vi "Pump_statusrequest.vi"(8 "error in (no error)":errorcluster, 10 "Command":string, 11 "VISA resource name":refnum<visa-resource-name>) -> (0 "error out":errorcluster, 1 "Message":string, 2 "Ready":bool, 3 "VISA resource name Out":refnum<visa-resource-name>, 4 "unsigned byte array":u8[](array[numeric]), 6 "Boolean array":bool[](array[boolean]))   [LabVIEW 2024]
uses:
  ab3bbe5a-7c2c-441d-9bf7-38fddc6173b4.vi
panel:
  out "Error present":bool
  out "read buffer":string
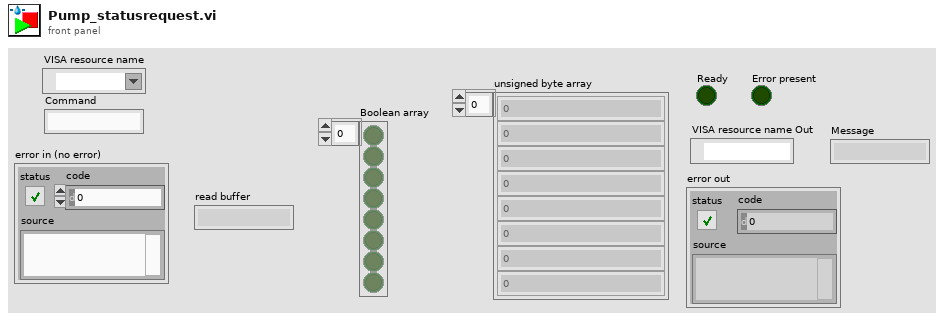
[diagram p1: front panel]
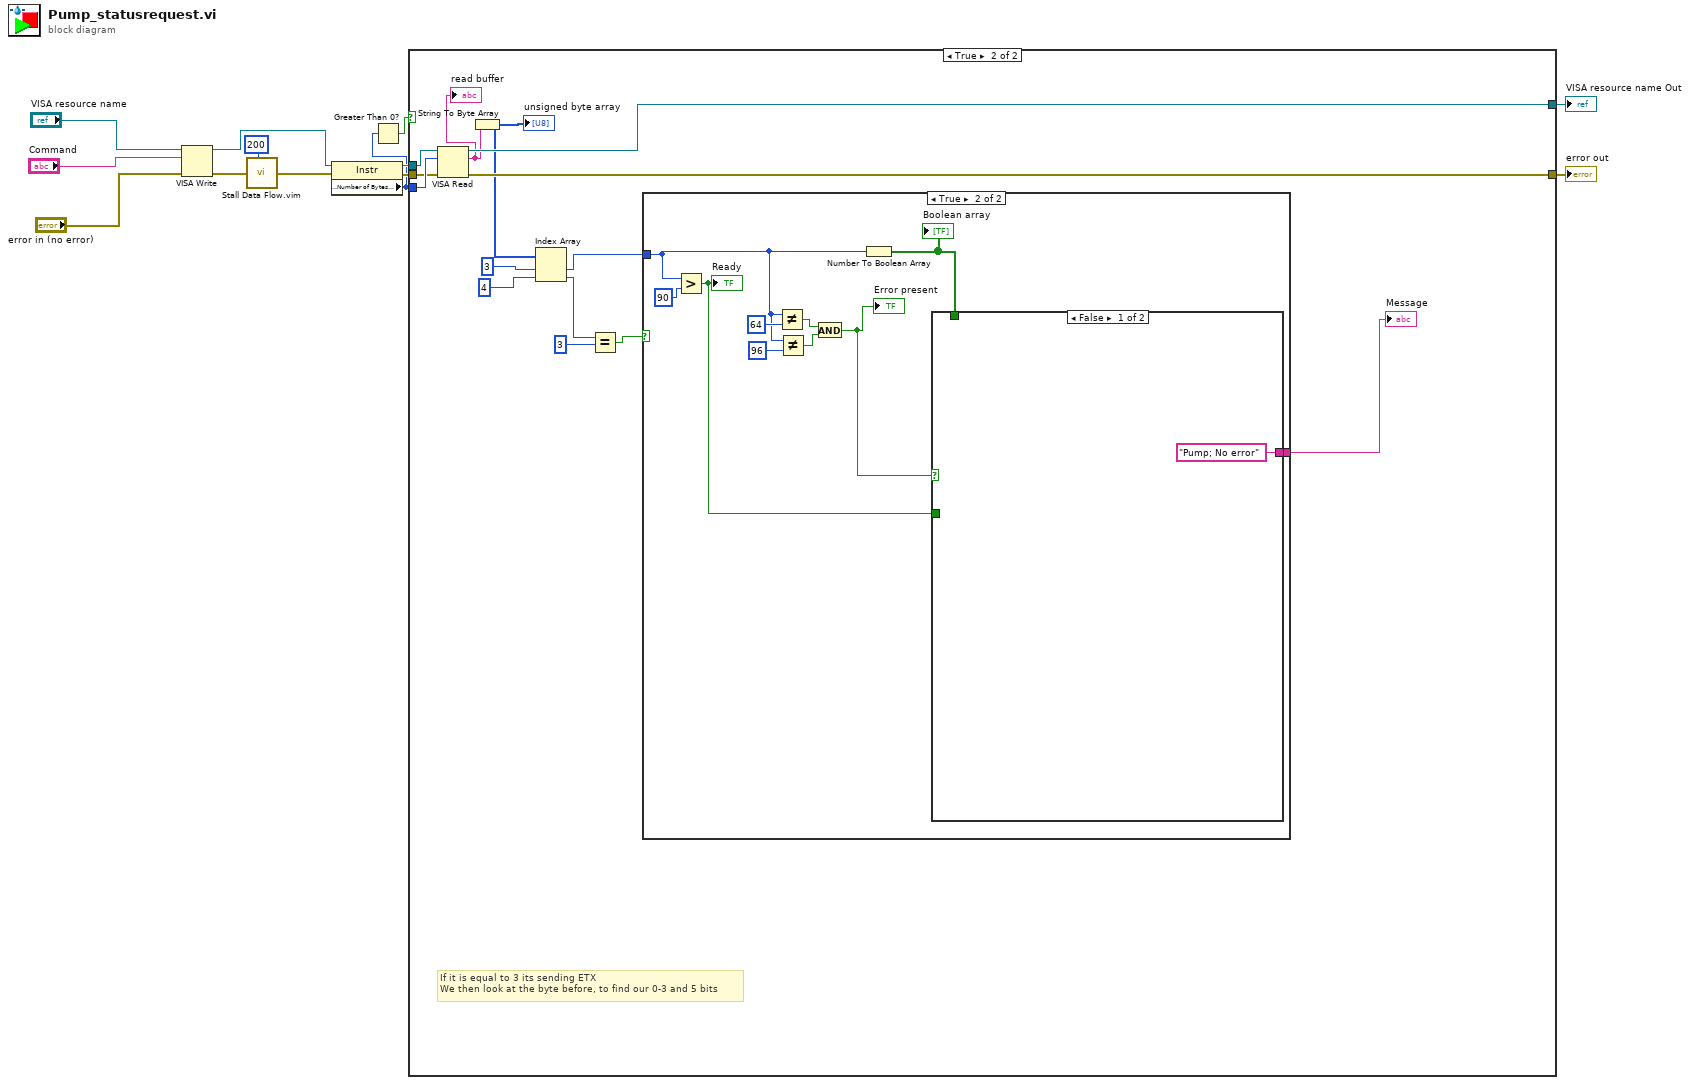
[diagram p0: block diagram]
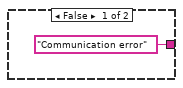
[diagram p3: hidden frame]
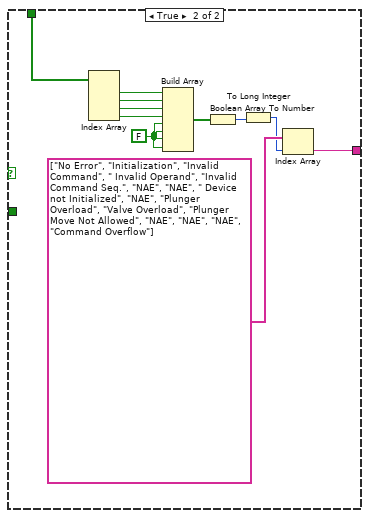
[diagram p4: hidden frame]
diagram:
  n1 = VISA Write(VISA resource name="VISA resource name", write buffer="Command", error in (no error)="error in (no error)") -> (VISA resource name out=w10:refnum<visa-resource-name>, error out=w13:errorcluster)  [unwired: 1 out]
  n2 = call "Stall Data Flow.vim"("value in"=w13, "milliseconds to wait"=u32 200) -> ("value out"=w11:errorcluster)  [unwired: 1 out]
  n3 = property class="Instr"(reference=w10, error in=w11) -> (reference out=w8:refnum<visa-resource-name>, error out=w9:errorcluster, "Serial Settings:Number of Bytes at Serial Port"=w7:u32)
  n4 = Greater Than 0?(x=w7) -> (x > 0?=w6:bool)
  n5 = case shown="True" w6 {
    tunnel: [w15 w29] -> w1
    tunnel: [w14 w28] -> w2
    tunnel: w7 -> [_ w19]
    tunnel: w9 -> [w14 w18]
    tunnel: w8 -> [w15 w17]
    frame False {
    }
    frame True {
      # "If it is equal to 3 its sending ETX\nWe then look at the byte before, to find our 0-3 and 5 bits"
      n6 = VISA Read(VISA resource name=w17, byte count=w19, error in (no error)=w18) -> (VISA resource name out=w29:refnum<visa-resource-name>, read buffer=w27:string, error out=w28:errorcluster)  [unwired: 1 out]
      "read buffer" <- w27
      n7 = String To Byte Array(string=w27) -> (unsigned byte array=w26:u8[])
      "unsigned byte array" <- w26
      n8 = Index Array(array=w26, index #1=3 ("index"), index #2=4 ("index")) -> (element #1=w20:u8, element #2=w22:u8)
      n9 = Equal?(x=w22, y=u8 3 ("x")) -> (x = y?=w21:bool)
      n10 = case shown="True" w21 {
        tunnel: w20 -> [_ w33]
        tunnel: ["Communication error" w31] -> w16
        frame False {
        }
        frame True {
          n11 = Greater?(x=w33, y=u8 90) -> (0:w34:bool)
          "Ready" <- w34
          n12 = Not Equal?(x=w33, y=u8 64) -> (x != y?=w37:bool)
          n13 = Not Equal?(x=w33, y=u8 96) -> (x != y?=w36:bool)
          n14 = And(x=w37, y=w36) -> (x .and. y?=w35:bool)
          "Error present" <- w35
          n15 = Number To Boolean Array(number=w33) -> (Boolean array=w32:bool[])
          "Boolean array" <- w32
          n16 = case shown="False" w35 {
            tunnel: w34 -> [_ _]
            tunnel: w32 -> [_ w52]
            tunnel: ["Pump; No error" w42] -> w31
            frame False {
            }
            frame True {
              w47 = FALSE
              n17 = Index Array(array=w52) -> (element #1=w51:bool, element #2=w50:bool, element #3=w49:bool, element #4=w48:bool)  [unwired: 4 in]
              n18 = Build Array(w51, w50, w49, w48, w47, w47, w47, w47) -> (w46:bool[])
              n19 = Boolean Array To Number(Boolean array=w46) -> (number=w44:u32)
              n20 = To Long Integer(number=w44) -> (32bit integer=w43:i32)
              n21 = Index Array(array=string[] ["No Error", "Initialization", "Invalid Command", " Invalid Operand", "Invalid Command Seq.", "NAE", "NAE", " Device not Initialized", "NAE", "Plunger Overload", "Valve Overload", "Plunger Move Not Allowed", "NAE", "NAE", "NAE", "Command Overflow"], index=w43) -> (element=w42:string)
            }
          }
        }
      }
      "Message" <- w16
    }
  }
  "error out" <- w2
  "VISA resource name Out" <- w1
